vi "MotorWaitEjeY_V3.vi"(8 "error in (no error)":errorcluster, 10 "Valor":dbl, 11 "CU ID":i32) -> (0 "error out":errorcluster)   [LabVIEW 2020]
panel:
  out "Error":dbl
  in  "Tolerance":dbl=0.0006
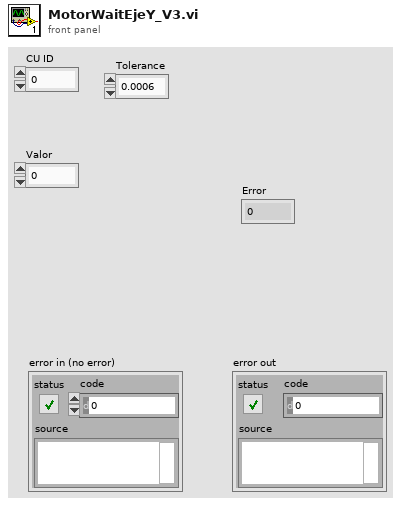
[diagram p1: front panel]
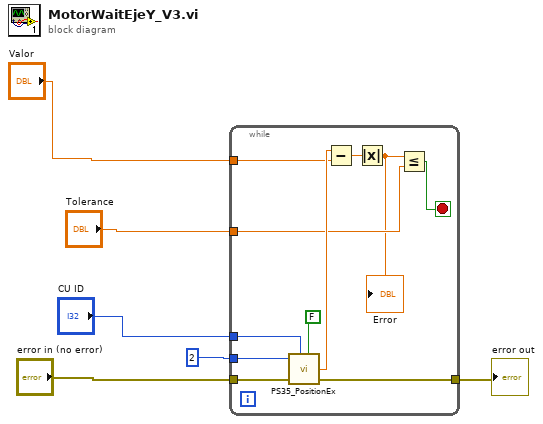
[diagram p0: block diagram]
diagram:
  n1 = while {
    tunnel: 2 -> [w16]
    tunnel: "CU ID" -> [w17]
    tunnel: "error in (no error)" -> [w14]
    tunnel: [w12] -> w6
    tunnel: "Valor" -> [w11]
    tunnel: "Tolerance" -> [w9]
    stop <- w10 stop-if-true
    n2 = call "PS35_PositionEx.vi"("Axis number"=w16, "Control unit ID"=w17, "error in (no error)"=w14, "function"=FALSE) -> ("dValue-Out"=w13:dbl, "error out"=w12:errorcluster)  [unwired: 4 in]
    n3 = Subtract(x=w13, y=w11) -> (x-y=w8:dbl)
    n4 = Absolute Value(x=w8) -> (abs(x)=w7:dbl)
    "Error" <- w7
    n5 = Less Or Equal?(x=w7, y=w9) -> (x <= y?=w10:bool)
  }
  "error out" <- w6
